vi "initArray.vi"() -> (0 "initialized array":i32[][](array[numeric]))   [LabVIEW 2013]
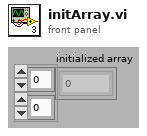
[diagram p1: front panel]
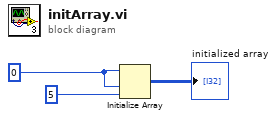
[diagram p0: block diagram]
diagram:
  w2 = 0
  n1 = Initialize Array(w2, w2, 5) -> (→"initialized array":i32[][])
